vi "Get Profile Header-Footer Size.vi"() -> (0 "Footer Size(DWORD)":u32, 1 "Header Size(DWORD)":u32, 2 "Footer Size(Byte)":u32, 3 "Header Size(Byte)":u32)   [LabVIEW 2020, in "KEYENCE LJ-X8000A.lvlib"]
uses:
  KEYENCE LJ-X8000A.lvlib
  Public/Clusters/Profile Header.ctl
  Public/Clusters/Profile Footer.ctl
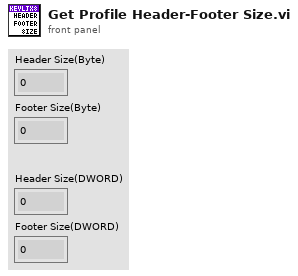
[diagram p1: front panel]
types:
  T1 = typedef "KEYENCE LJ-X8000A.lvlib/Profile Footer.ctl" = cluster{"reserve":u32}
  T2 = typedef "KEYENCE LJ-X8000A.lvlib/Profile Header.ctl" = cluster{"Encoder Z-in":u32, "Trigger Cnt":u32, "Encoder Cnt":u32, "reserve":u32, "reserve":u32, "reserve":u32}
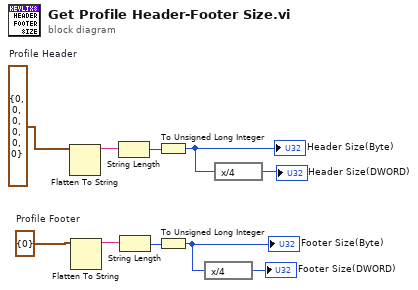
[diagram p0: block diagram]
diagram:
  w6 = T1 {"reserve"=0}  # Profile Footer
  w5 = T2 {"Encoder Z-in"=0, "Trigger Cnt"=0, "Encoder Cnt"=0, "reserve"=0, "reserve"=0, "reserve"=0}  # Profile Header
  n1 = Flatten To String(anything=w5) -> (data string=w10:string)  [unwired: 3 in, 2 out]
  n2 = Flatten To String(anything=w6) -> (data string=w9:string)  [unwired: 3 in, 2 out]
  n3 = String Length(string=w10) -> (length=w8:i32)
  n4 = String Length(string=w9) -> (length=w7:i32)
  n5 = To Unsigned Long Integer(number=w8) -> (unsigned 32bit integer=w4:u32)
  "Header Size(Byte)" <- w4
  n6 = To Unsigned Long Integer(number=w7) -> (unsigned 32bit integer=w2:u32)
  "Footer Size(Byte)" <- w2
  n7 = expression code="x/4"(w2) -> (→"Footer Size(DWORD)":u32)
  n8 = expression code="x/4"(w4) -> (→"Header Size(DWORD)":u32)
